vi "dvr_fgv_map.vi"(8 "error in (no error)":errorcluster) -> (0 "error out":errorcluster, 3 "data value reference":refnum<data-value>)   [LabVIEW 2020]
uses:
  map_state.ctl
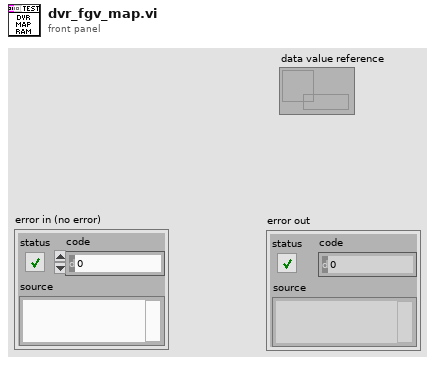
[diagram p1: front panel]
types:
  T1 = typedef "map_state.ctl" = enum16{"flag"}
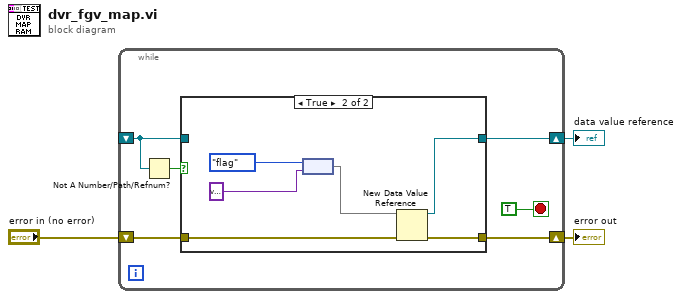
[diagram p0: block diagram]
diagram:
  n1 = while {
    shift-right: [w7] -> w2
    shift-left: "error in (no error)" -> [w8]
    shift-right: [w6] -> w1
    shift-left: _ -> [w4]
    stop <- TRUE stop-if-true
    n2 = Not A Number/Path/Refnum?(number/path/refnum=w4) -> (NaN/Path/Refnum?=w5:bool)
    n3 = case shown="True" w5 {
      tunnel: w8 -> [w10 w14]
      tunnel: [w10 w13] -> w7
      tunnel: [w11 w12] -> w6
      tunnel: w4 -> [w11 _]
      frame False {
      }
      frame True {
        n4 = node(map_state."flag", variant) -> (w15:map{T1, variant})
        n5 = New Data Value Reference(data value=w15, error in=w14) -> (data value reference=w12:refnum<data-value>, error out=w13:errorcluster)
      }
    }
  }
  "error out" <- w2
  "data value reference" <- w1
